vi "Get User Items.vi"(10 "USER/ITEM DATA TRANSFER":T2(array[cluster]), 11 "REFERENCES":T1) -> ()   [LabVIEW 2019]
uses:
  Controls/References Cluster.ctl
  Controls/Custom Calendar/Custom Calendar.xctl
  <vilib>/addons/database/Auxilliary.llb/DB Tools Cursor Type.ctl
  <vilib>/Utility/miscctls.llb/LVRowAndColumnTypeDef.ctl
  Controls/Column Names/Inventory Column Names.ctl
  <vilib>/addons/database/Connection.llb/DB Tools Open Connec (String).vi
  <vilib>/addons/database/Connection.llb/Conn Execute.vi
  <vilib>/addons/database/Recordset.llb/Rec Fetch Recordset Data (R).vi
  <vilib>/addons/database/Recordset.llb/Rec Destroy - Connection.vi
  <vilib>/addons/database/_DB Variant To Data/Database Variant To Data.xnode
  <vilib>/addons/database/NI_Database_API.lvlib
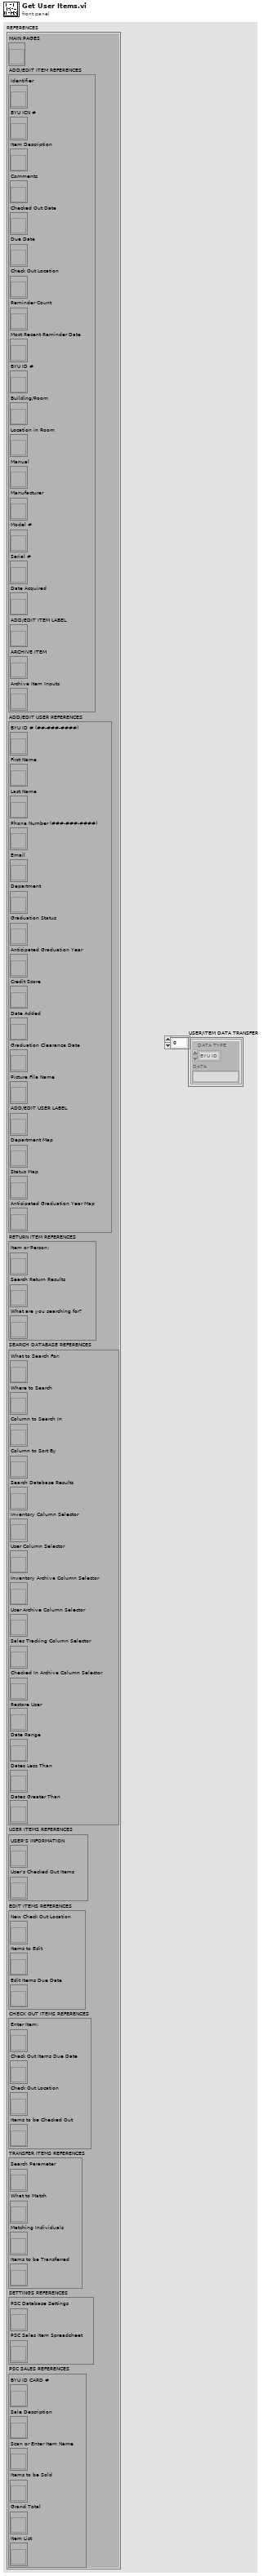
[diagram p1: front panel]
types:
  T1 = typedef "References Cluster.ctl" = cluster{"MAIN PAGES":refnum<vi>, "ADD/EDIT ITEM REFERENCES":cluster{"Identifier":refnum<vi>, "BYU ICN #":refnum<vi>, "Item Description":refnum<vi>, "Comments":refnum<vi>, "Checked Out Date":refnum<vi>, "Due Date":refnum<vi>, "Check Out Location":refnum<vi>, "Reminder Count":refnum<vi>, "Most Recent Reminder Date":refnum<vi>, "BYU ID #":refnum<vi>, "Building/Room":refnum<vi>, "Location in Room":refnum<vi>, "Manual":refnum<vi>, "Manufacturer":refnum<vi>, "Model #":refnum<vi>, "Serial #":refnum<vi>, "Date Acquired":refnum<vi>, "ADD/EDIT ITEM LABEL":refnum<vi>, "ARCHIVE ITEM":refnum<vi>, "Archive Item Inputs":refnum<vi>}, "ADD/EDIT USER REFERENCES":cluster{"BYU ID # (##-###-####)":refnum<vi>, "First Name":refnum<vi>, "Last Name":refnum<vi>, "Phone Number (###-###-####)":refnum<vi>, "Email":refnum<vi>, "Department":refnum<vi>, "Graduation Status":refnum<vi>, "Anticipated Graduation Year":refnum<vi>, "Credit Score":refnum<vi>, "Date Added":refnum<vi>, "Graduation Clearance Date":refnum<vi>, "Picture File Name":refnum<vi>, "ADD/EDIT USER LABEL":refnum<vi>, "Department Map":refnum<vi>, "Status Map":refnum<vi>, "Anticipated Graduation Year Map":refnum<vi>}, "RETURN ITEM REFERENCES":cluster{"Item or Person:":refnum<vi>, "Search Return Results":refnum<vi>, "What are you searching for?":refnum<vi>}, "SEARCH DATABASE REFERENCES":cluster{"What to Search For:":refnum<vi>, "Where to Search":refnum<vi>, "Column to Search In":refnum<vi>, "Column to Sort By":refnum<vi>, "Search Database Results":refnum<vi>, "Inventory Column Selector":refnum<vi>, "User Column Selector":refnum<vi>, "Inventory Archive Column Selector":refnum<vi>, "User Archive Column Selector":refnum<vi>, "Sales Tracking Column Selector":refnum<vi>, "Checked In Archive Column Selector":refnum<vi>, "Restore User":refnum<vi>, "Date Range":refnum<vi>, "Dates Less Than":refnum<vi>, "Dates Greater Than":refnum<vi>}, "USER ITEMS REFERENCES":cluster{"USER'S INFORMATION":refnum<vi>, "User's Checked Out Items":refnum<vi>}, "EDIT ITEMS REFERENCES":cluster{"New Check Out Location":refnum<vi>, "Items to Edit":refnum<vi>, "Edit Items Due Date":refnum<vi>}, "CHECK OUT ITEMS REFERENCES":cluster{"Enter Item:":refnum<vi>, "Check Out Items Due Date":refnum<vi>, "Check Out Location":refnum<vi>, "Items to be Checked Out":refnum<vi>}, "TRANSFER ITEMS REFERENCES":cluster{"Search Parameter":refnum<vi>, "What to Match":refnum<vi>, "Matching Individuals":refnum<vi>, "Items to be Transferred":refnum<vi>}, "SETTINGS REFERENCES":cluster{"PSC Database Settings":refnum<vi>, "PSC Sales Item Spreadsheet":refnum<vi>}, "PSC SALES REFERENCES":cluster{"BYU ID CARD #":refnum<vi>, "Sale Description":refnum<vi>, "Scan or Enter Item Name":refnum<vi>, "Items to be Sold":refnum<vi>, "Grand Total":refnum<vi>, "Item List":refnum<vi>}}
  T2 = cluster{"DATA TYPE":enum16{"BYU ID", "ME#/IDENTIFIER", "BYU ICN"}, "DATA":string}[]
  T3 = typedef "Inventory Column Names.ctl" = string[]
  T4 = typedef "LVRowAndColumnTypeDef.ctl" = cluster{"Row":i32, "Column":i32}
  T5 = typedef "NI_Database_API.lvlib/DB Tools Cursor Type.ctl" = enum16{"forward-only", "keyset", "dynamic", "static"}
  T6 = cluster{"DATA TYPE":enum16{"BYU ID", "ME#/IDENTIFIER", "BYU ICN"}, "DATA":string}
  T7 = cluster{"USER'S INFORMATION":refnum<vi>, "User's Checked Out Items":refnum<vi>}
  T8 = typedef "NI_Database_API.lvlib/Conn ObjectReference.ctl" = refnum<k1>
  T9 = typedef "NI_Database_API.lvlib/Rec ObjectReference.ctl" = refnum<k1>
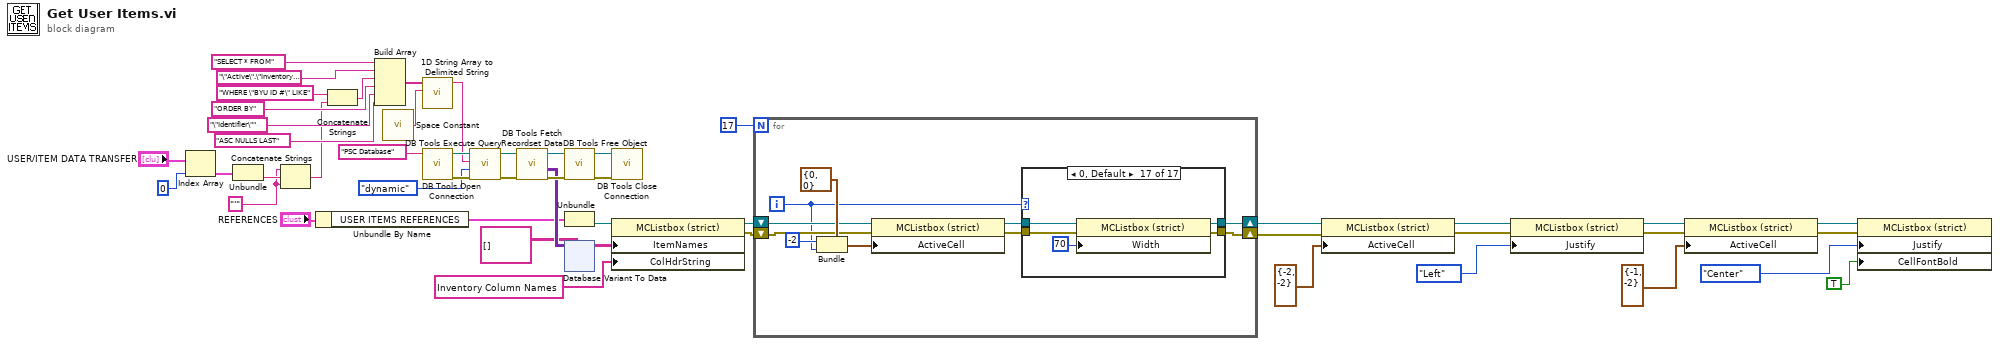
[diagram p0: block diagram]
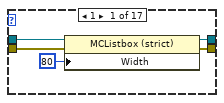
[diagram p2: hidden frame]
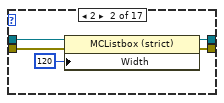
[diagram p3: hidden frame]
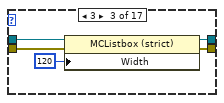
[diagram p4: hidden frame]
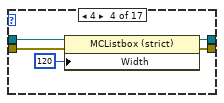
[diagram p5: hidden frame]
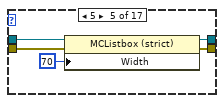
[diagram p6: hidden frame]
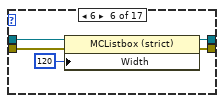
[diagram p7: hidden frame]
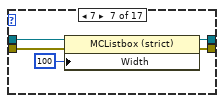
[diagram p8: hidden frame]
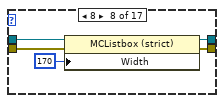
[diagram p9: hidden frame]
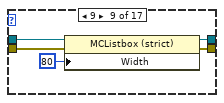
[diagram p10: hidden frame]
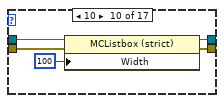
[diagram p11: hidden frame]
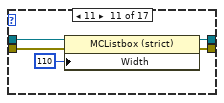
[diagram p12: hidden frame]
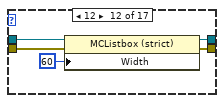
[diagram p13: hidden frame]
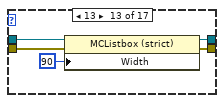
[diagram p14: hidden frame]
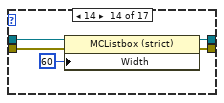
[diagram p15: hidden frame]
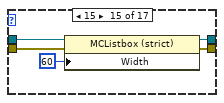
[diagram p16: hidden frame]
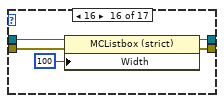
[diagram p17: hidden frame]
diagram:
  w18 = "'"
  n1 = Index Array(array="USER/ITEM DATA TRANSFER", index=0) -> (element=w27:T6)
  n2 = Unbundle(w27) -> ("DATA"=w19:string)  [unwired: 1 out]
  n3 = Concatenate Strings(w18, w19, w18) -> (w20:string)
  n4 = Unbundle By Name("REFERENCES") -> ("USER ITEMS REFERENCES"=w24:T7)
  n5 = Concatenate Strings("WHERE \"BYU ID #\" LIKE", w20) -> (w44:string)
  n6 = Build Array("SELECT * FROM", "\"Active\".\"Inventory\"", w44, "ORDER BY", "\"Identifier\"", "ASC NULLS LAST") -> (w42:string[])
  n7 = call <vilib>:"Space Constant.vi"() -> ("String"=w41:string)
  n8 = call <vilib>:"1D String Array to Delimited String.vi"("delimiter"=w41, "string array"=w42) -> ("delimited string"=w40:string)  [unwired: 9 in]
  n9 = call-poly <vilib>:"DB Tools Open Connection.vi"("connection information"="PSC Database") -> ("error out"=w47:errorcluster, "connection reference"=w49:T8)  [unwired: 7 in]
  n10 = call-poly <vilib>:"DB Tools Execute Query.vi"("error in (no error)"=w47, "cursor type"=DB_Tools_Cursor_Type."dynamic", "SQL query"=w40, "connection reference"=w49) -> ("error out"=w37:errorcluster, "recordset reference"=w38:T9)  [unwired: 4 in]
  n11 = call-poly <vilib>:"DB Tools Fetch Recordset Data.vi"("error in (no error)"=w37, "recordset reference"=w38) -> ("error out"=w35:errorcluster, "recordset data"=w32:variant[][], "recordset reference out"=w36:T9)  [unwired: 3 in]
  n12 = call-poly <vilib>:"DB Tools Free Object.vi"("error in (no error)"=w35, "recordset reference"=w36) -> ("error out"=w33:errorcluster, "connection reference"=w34:T8)  [unwired: 8 in]
  n13 = Unbundle(w24) -> ("User's Checked Out Items"=w31:refnum<vi>)  [unwired: 1 out]
  n14 = xnode "Database Variant To Data"("database variant"=w32, "type"=string[][] []) -> ("data"=w23:string[][])  [unwired: 1 in, 1 out]
  n15 = call <vilib>:"DB Tools Close Connection.vi"("error in (no error)"=w33, "connection reference"=w34) -> ()  [unwired: 5 in, 1 out]
  n16 = property class="MCListbox (strict)"(reference=w31, "ItemNames"=w23, "ColHdrString"=T3 ["ME #/ID #", "BYU ICN #", "Item Description", "Comments", "Checked Out Date", "Due Date", "Check Out Location", "Reminder Count", "Most Recent Reminder Date", "BYU ID #", "Building/Room", "Location in Room", "Manual", "Manufacturer", "Model #", "Serial #", "Date Acquired"] ("INVENTORY COLUMN NAMES")) -> (reference out=w6:refnum<vi>, error out=w5:errorcluster)  [unwired: 1 in]
  n17 = for {
    N: 17 -> [_]
    shift-right: [w54] -> w3
    shift-left: w6 -> [w56]
    shift-right: [w51] -> w2
    shift-left: w5 -> [w53]
    i -> [w50]
    n18 = Bundle(cluster=T4 {"Row"=0, "Column"=0} ("Active Cell:Active Cell"), "Row"=-2, "Column"=w50) -> (w58:T4)
    n19 = property class="MCListbox (strict)"(reference=w56, error in=w53, "ActiveCell"=w58) -> (reference out=w57:refnum<vi>, error out=w52:errorcluster)
    n20 = case shown="0, Default" w50 {
      tunnel: w57 -> [w64 w69 w74 w79 w84 w89 w94 w99 w104 w109 w114 w119 w124 w129 w134 w139 w144]
      tunnel: [w62 w67 w72 w77 w82 w87 w92 w97 w102 w107 w112 w117 w122 w127 w132 w137 w142] -> w54
      tunnel: w52 -> [w61 w66 w71 w76 w81 w86 w91 w96 w101 w106 w111 w116 w121 w126 w131 w136 w141]
      tunnel: [w60 w65 w70 w75 w80 w85 w90 w95 w100 w105 w110 w115 w120 w125 w130 w135 w140] -> w51
      frame 1 {
        n21 = property class="MCListbox (strict)"(reference=w64, error in=w61, "Width"=u32 80 ("Active Cell:Cell Size:Width")) -> (reference out=w62:refnum<vi>, error out=w60:errorcluster)
      }
      frame 2 {
        n22 = property class="MCListbox (strict)"(reference=w69, error in=w66, "Width"=u32 120 ("Active Cell:Cell Size:Width")) -> (reference out=w67:refnum<vi>, error out=w65:errorcluster)
      }
      frame 3 {
        n23 = property class="MCListbox (strict)"(reference=w74, error in=w71, "Width"=u32 120 ("Active Cell:Cell Size:Width")) -> (reference out=w72:refnum<vi>, error out=w70:errorcluster)
      }
      frame 4 {
        n24 = property class="MCListbox (strict)"(reference=w79, error in=w76, "Width"=u32 120 ("Active Cell:Cell Size:Width")) -> (reference out=w77:refnum<vi>, error out=w75:errorcluster)
      }
      frame 5 {
        n25 = property class="MCListbox (strict)"(reference=w84, error in=w81, "Width"=u32 70 ("Active Cell:Cell Size:Width")) -> (reference out=w82:refnum<vi>, error out=w80:errorcluster)
      }
      frame 6 {
        n26 = property class="MCListbox (strict)"(reference=w89, error in=w86, "Width"=u32 120 ("Active Cell:Cell Size:Width")) -> (reference out=w87:refnum<vi>, error out=w85:errorcluster)
      }
      frame 7 {
        n27 = property class="MCListbox (strict)"(reference=w94, error in=w91, "Width"=u32 100 ("Active Cell:Cell Size:Width")) -> (reference out=w92:refnum<vi>, error out=w90:errorcluster)
      }
      frame 8 {
        n28 = property class="MCListbox (strict)"(reference=w99, error in=w96, "Width"=u32 170 ("Active Cell:Cell Size:Width")) -> (reference out=w97:refnum<vi>, error out=w95:errorcluster)
      }
      frame 9 {
        n29 = property class="MCListbox (strict)"(reference=w104, error in=w101, "Width"=u32 80 ("Active Cell:Cell Size:Width")) -> (reference out=w102:refnum<vi>, error out=w100:errorcluster)
      }
      frame 10 {
        n30 = property class="MCListbox (strict)"(reference=w109, error in=w106, "Width"=u32 100 ("Active Cell:Cell Size:Width")) -> (reference out=w107:refnum<vi>, error out=w105:errorcluster)
      }
      frame 11 {
        n31 = property class="MCListbox (strict)"(reference=w114, error in=w111, "Width"=u32 110 ("Active Cell:Cell Size:Width")) -> (reference out=w112:refnum<vi>, error out=w110:errorcluster)
      }
      frame 12 {
        n32 = property class="MCListbox (strict)"(reference=w119, error in=w116, "Width"=u32 60 ("Active Cell:Cell Size:Width")) -> (reference out=w117:refnum<vi>, error out=w115:errorcluster)
      }
      frame 13 {
        n33 = property class="MCListbox (strict)"(reference=w124, error in=w121, "Width"=u32 90 ("Active Cell:Cell Size:Width")) -> (reference out=w122:refnum<vi>, error out=w120:errorcluster)
      }
      frame 14 {
        n34 = property class="MCListbox (strict)"(reference=w129, error in=w126, "Width"=u32 60 ("Active Cell:Cell Size:Width")) -> (reference out=w127:refnum<vi>, error out=w125:errorcluster)
      }
      frame 15 {
        n35 = property class="MCListbox (strict)"(reference=w134, error in=w131, "Width"=u32 60 ("Active Cell:Cell Size:Width")) -> (reference out=w132:refnum<vi>, error out=w130:errorcluster)
      }
      frame 16 {
        n36 = property class="MCListbox (strict)"(reference=w139, error in=w136, "Width"=u32 100 ("Active Cell:Cell Size:Width")) -> (reference out=w137:refnum<vi>, error out=w135:errorcluster)
      }
      frame 0, Default {
        n37 = property class="MCListbox (strict)"(reference=w144, error in=w141, "Width"=u32 70 ("Active Cell:Cell Size:Width")) -> (reference out=w142:refnum<vi>, error out=w140:errorcluster)
      }
    }
  }
  n38 = property class="MCListbox (strict)"(reference=w3, error in=w2, "ActiveCell"=T4 {"Row"=-2, "Column"=-2} ("Active Cell:Active Cell")) -> (reference out=w16:refnum<vi>, error out=w15:errorcluster)
  n39 = property class="MCListbox (strict)"(reference=w16, error in=w15, "Justify"=enum16{"Left", "Center", "Right"}."Left" ("Active Cell:Cell Justification")) -> (reference out=w11:refnum<vi>, error out=w10:errorcluster)
  n40 = property class="MCListbox (strict)"(reference=w11, error in=w10, "ActiveCell"=T4 {"Row"=-1, "Column"=-2} ("Active Cell:Active Cell")) -> (reference out=w12:refnum<vi>, error out=w13:errorcluster)
  n41 = property class="MCListbox (strict)"(reference=w12, error in=w13, "Justify"=enum16{"Left", "Center", "Right"}."Center" ("Active Cell:Cell Justification"), "CellFontBold"=TRUE ("Active Cell:Cell Font:Bold")) -> ()  [unwired: 2 out]
